vi "Reporting_proc_inycom.vi"(2 "cluster":cluster{i64[], bool}, 3 "address repoting":path) -> (1 "Reporting":string)   [LabVIEW 2015]
panel:
  out "error out":errorcluster
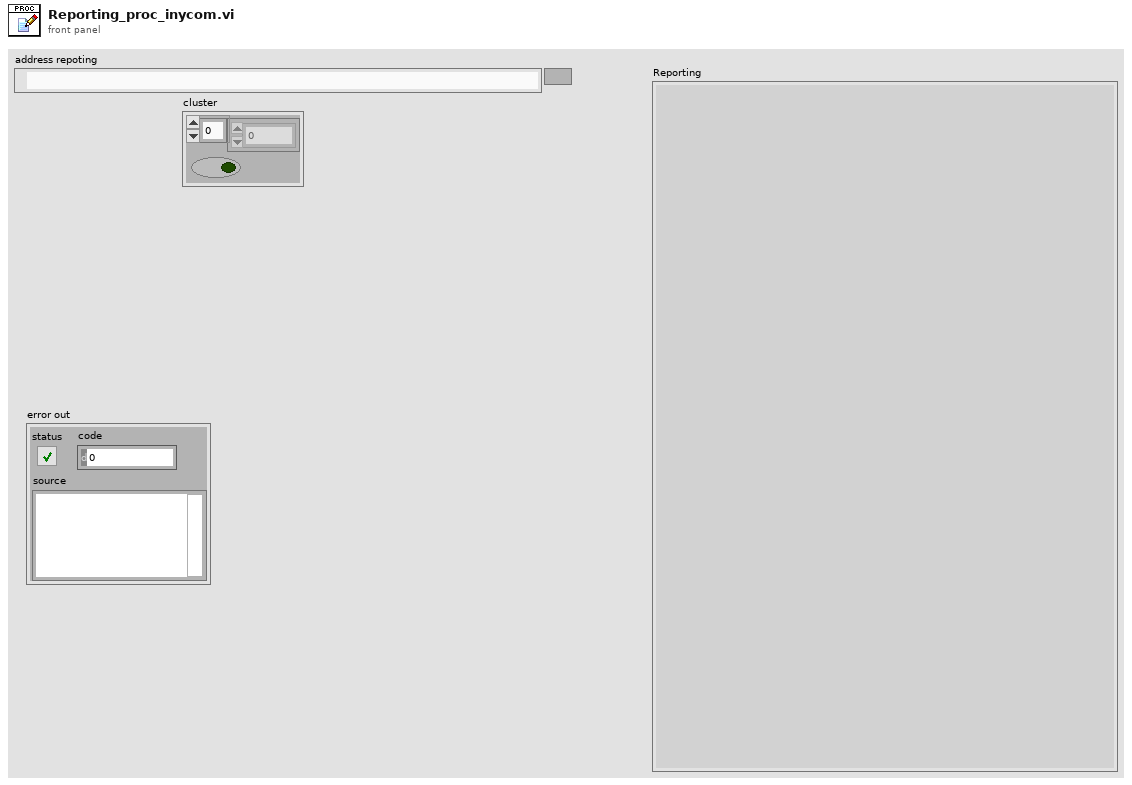
[diagram p1: front panel]
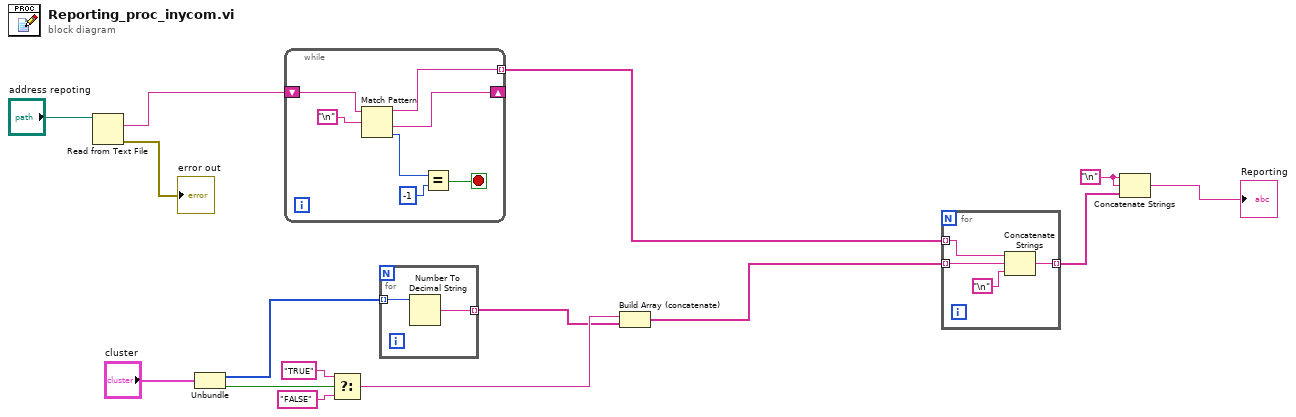
[diagram p0: block diagram]
diagram:
  w10 = "\n"
  n1 = Read from Text File(file (use dialog)="address repoting") -> (text=w15:string, error out=→"error out":errorcluster)  [unwired: 3 in, 2 out]
  n2 = Unbundle("cluster") -> (w5:i64[], w7:bool)
  n3 = while {
    tunnel: [w19] -> w4 mode=indexing
    shift-right: [w16] -> _
    shift-left: w15 -> [w17]
    stop <- w22 stop-if-true
    n4 = Match Pattern(string=w17, regular expression="\n") -> (before substring=w19:string, after substring=w16:string, offset past match=w20:i32)  [unwired: 1 in, 1 out]
    n5 = Equal?(x=w20, y=-1) -> (x = y?=w22:bool)
  }
  n6 = Select(t="TRUE", s=w7, f="FALSE") -> (s? t:f=w3:string)
  n7 = for {
    tunnel: w5 -> [w24] mode=indexing
    tunnel: [w23] -> w2 mode=indexing
    n8 = Number To Decimal String(number=w24) -> (decimal integer string=w23:string)  [unwired: 1 in]
  }
  n9 = Build Array (concatenate)(w3, w2) -> (w1:string[])
  n10 = for {
    tunnel: [w27] -> w12 mode=indexing
    tunnel: w4 -> [w25] mode=indexing
    tunnel: w1 -> [w26] mode=indexing
    n11 = Concatenate Strings(w25, w26, "\n") -> (w27:string)
  }
  n12 = Concatenate Strings(w10, w10, w12) -> (→"Reporting":string)
